vi "Get All Sections.vi"(8 "error in":errorcluster, 11 "Item in":refnum<class "Item.lvclass">) -> (0 "error out":errorcluster, 2 "Sections out":refnum<class "Section.lvclass">[](array[class]), 3 "Item out":refnum<class "Item.lvclass">)   [LabVIEW 2024, in "Parser.lvlib" / "Section.lvclass"]
uses:
  Section.lvclass
  Item/Item.lvclass
  Item/Item.lvclass/Item.ctl
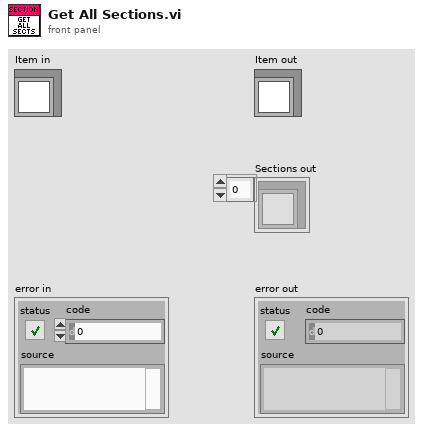
[diagram p1: front panel]
types:
  T1 = typedef "Parser.lvlib/Item.lvclass/Item Type.ctl" = enum16{"Channel", "Section"}
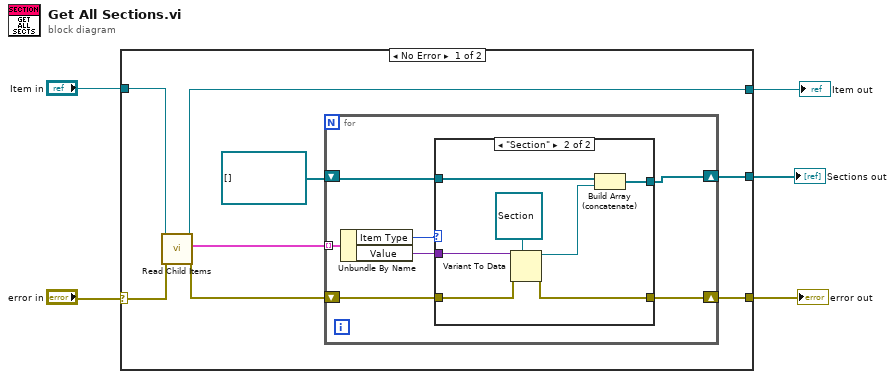
[diagram p0: block diagram]
diagram:
  n1 = case shown="No Error" "error in" {
    selector: "error in" -> [w11 w31]
    tunnel: [w12 w31] -> w5
    tunnel: "Item in" -> [w9 w30]
    tunnel: [w8 w30] -> w2
    tunnel: [w6 _] -> w1
    frame No Error {
      n2 = call "Read Child Items.vi"("error in"=w11, "Item in"=w9) -> ("error out"=w13:errorcluster, "Child Items"=w10:cluster{"Item Type":T1, "Value":variant}[], "Item out"=w8:refnum<class "Item.lvclass">)  [unwired: 7 in]
      n3 = for {
        tunnel: w10 -> [w18] mode=indexing
        shift-right: [w19] -> w12
        shift-left: w13 -> [w20]
        shift-right: [w14] -> w6
        shift-left: refnum<class "Section.lvclass">[] [] -> [w15]
        n4 = Unbundle By Name(w18) -> ("Item Type"=w17:T1, "Value"=w16:variant)
        n5 = case shown="\"Section\"" w17 {
          tunnel: w16 -> [_ w27]
          tunnel: w20 -> [w22 w29]
          tunnel: [w22 w28] -> w19
          tunnel: w15 -> [w21 w26]
          tunnel: [w21 w24] -> w14
          frame Default {
          }
          frame "Section" {
            n6 = Variant To Data(error in=w29, type=refnum<class "Section.lvclass"> refnum ("Section"), Variant=w27) -> (data=w25:refnum<class "Section.lvclass">, error out=w28:errorcluster)
            n7 = Build Array (concatenate)(w26, w25) -> (w24:refnum<class "Section.lvclass">[])
          }
        }
      }
    }
    frame Error {
    }
  }
  "error out" <- w5
  "Item out" <- w2
  "Sections out" <- w1
